vi "Intake Rollers.vi"   [LabVIEW 2014]
uses:
  <vilib>/Rock Robotics/WPI/Solenoid/WPI_SolenoidValue.ctl
  Begin/Global RefNums.vi
  Begin/Global Variables.vi
  <vilib>/Rock Robotics/WPI/Solenoid/WPI_SolenoidSetEnum.vi
types:
  T1 = typedef "WPI_SolenoidValue.ctl" = enum16{"Off", "On", "Forward", "Reverse"}
  T2 = typedef "WPI_MotorControlDeviceRef.ctl" = cluster{"DeviceStatus":errorcluster, "Type":T3, "PWM":cluster{"Controller":T4, "PWM Channel":T5, "DeadBand":T6}, "CAN":cluster{"Device Number":u8, "Control Mode":T7, "Semaphore":T8, "Max Vout":dbl, "TalonSRX Control Mode":T9}, "Invert":bool, "TransformRef":T10, "InvTransformRef":T10}
  T3 = typedef "WPI_MotorControlType.ctl" = enum16{"PWM", "CAN", "CANTalonSRX"}
  T4 = typedef "FPGA_TypedefDigitalModule.ctl" = enum16{"Controller 1"}
  T5 = typedef "FPGA_DIOPWMChannel.ctl" = enum8{"PWM 0", "PWM 1", "PWM 2", "PWM 3", "PWM 4", "PWM 5", "PWM 6", "PWM 7", "PWM 8", "PWM 9", "PWM MXP 0", "PWM MXP 1", "PWM MXP 2", "PWM MXP 3", "PWM MXP 4", "PWM MXP 5", "PWM MXP 6", "PWM MXP 7", "PWM MXP 8", "PWM MXP 9", "Invalid"}
  T6 = typedef "WPI_PWMDeadband.ctl" = cluster{"Name":string, "maxPositivePwm":i32, "minPositivePwm":i32, "centerPwm":i32, "maxNegativePwm":i32, "minNegativePwm":i32, "angularRange":u16}
  T7 = typedef "WPI_CANJaguar_ControlMode.ctl" = enum8{"Percent VBus", "Current", "Speed", "Position", "Voltage"}
  T8 = typedef "Semaphore RefNum" = refnum<k1>
  T9 = typedef "WPI_CANTalonSRX_APIControlMode.ctl" = enum8{"Percent VBus", "Speed", "Position", "Slave", "Unchanged / Invalid"}
  T10 = typedef "WPI_PWMTransform_ConPane.ctl" = refnum<vi>
  T11 = typedef "WPI_SolenoidDevRef.ctl" = cluster{"DevStatus":errorcluster, "Pneumatics Control Module":u8, "Forward Solenoid Channel":T12, "Reverse Solenoid Channel":T12}
  T12 = typedef "WPI_SolenoidChannel.ctl" = enum8{"Solenoid 0", "Solenoid 1", "Solenoid 2", "Solenoid 3", "Solenoid 4", "Solenoid 5", "Solenoid 6", "Solenoid 7", "Invalid"}
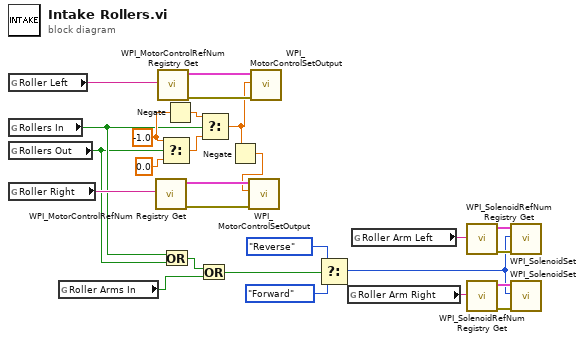
[diagram p0: block diagram]
diagram:
  w17 = -1.0 ("t")
  n1 = global read "Global RefNums.vi" "Roller Left"() -> (w24:string)
  n2 = global read "Global Variables.vi" "Rollers In"() -> (w14:bool)
  n3 = global read "Global Variables.vi" "Rollers Out"() -> (w13:bool)
  n4 = global read "Global RefNums.vi" "Roller Right"() -> (w23:string)
  n5 = global read "Global Variables.vi" "Roller Arms In"() -> (w11:bool)
  n6 = call <vilib>:"WPI_MotorControlRefNum Registry Get.vi"("refnum name"=w23) -> ("error out"=w21:errorcluster, "MotorControlDevRef"=w22:T2)  [unwired: 9 in]
  n7 = call <vilib>:"WPI_MotorControlRefNum Registry Get.vi"("refnum name"=w24) -> ("error out"=w26:errorcluster, "MotorControlDevRef"=w25:T2)  [unwired: 9 in]
  n8 = Select(t=w17, s=w13, f=0.0) -> (s? t:f=w20:dbl)
  n9 = Or(x=w14, y=w13) -> (x .or. y?=w12:bool)
  n10 = Negate(x=w17) -> (-x=w18:dbl)
  n11 = Or(x=w12, y=w11) -> (x .or. y?=w8:bool)
  n12 = Select(t=w18, s=w14, f=w20) -> (s? t:f=w16:dbl)
  n13 = Negate(x=w16) -> (-x=w15:dbl)
  n14 = call <vilib>:"WPI_MotorControlSetOutput.vi"("error in (no error)"=w21, "Output"=w15, "MotorControlDevRef"=w22) -> ()  [unwired: 6 in, 3 out]
  n15 = call <vilib>:"WPI_MotorControlSetOutput.vi"("error in (no error)"=w26, "Output"=w16, "MotorControlDevRef"=w25) -> ()  [unwired: 6 in, 3 out]
  n16 = Select(t=WPI_SolenoidValue."Reverse" ("Value"), s=w8, f=WPI_SolenoidValue."Forward" ("Value")) -> (s? t:f=w1:T1)
  n17 = global read "Global RefNums.vi" "Roller Arm Right"() -> (w4:string)
  n18 = global read "Global RefNums.vi" "Roller Arm Left"() -> (w5:string)
  n19 = call <vilib>:"WPI_SolenoidRefNum Registry Get.vi"("refnum name"=w5) -> ("error out"=w7:errorcluster, "SolenoidDevRef"=w6:T11)  [unwired: 9 in]
  n20 = call <vilib>:"WPI_SolenoidRefNum Registry Get.vi"("refnum name"=w4) -> ("error out"=w2:errorcluster, "SolenoidDevRef"=w3:T11)  [unwired: 9 in]
  n21 = call-poly <vilib>:"WPI_SolenoidSet.vi"("error in (no error)"=w7, "Value"=w1, "SolenoidDevRef"=w6) -> ()  [unwired: 7 in, 2 out]
  n22 = call-poly <vilib>:"WPI_SolenoidSet.vi"("error in (no error)"=w2, "Value"=w1, "SolenoidDevRef"=w3) -> ()  [unwired: 7 in, 2 out]
